vi "core_wait (global variable).vi"() -> ()   [LabVIEW 2020, in "core.lvlib"]
uses:
  core.lvlib
panel:
  in  "core_wait (ms)":u32
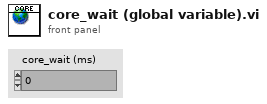
[diagram p1: front panel]
diagram:
